vi "JSONtoLV-DBInsert.vi"(8 "error in":errorcluster, 11 "Output JSON Object":string) -> (0 "error out":errorcluster, 3 "value":T1)   [LabVIEW 2013]
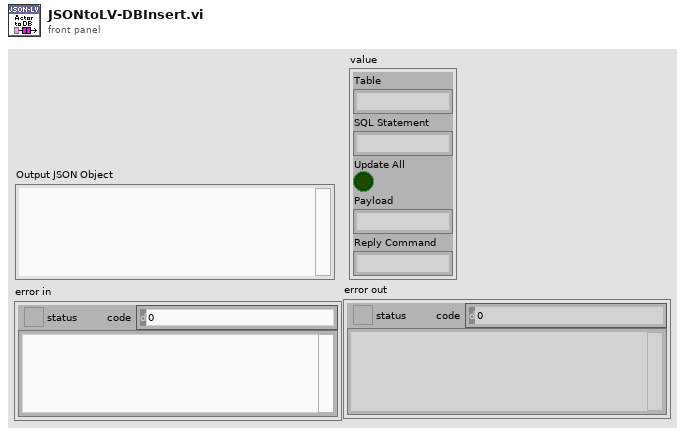
[diagram p1: front panel]
types:
  T1 = cluster{"Table":string, "SQL Statement":string, "Update All":bool, "Payload":string, "Reply Command":string}
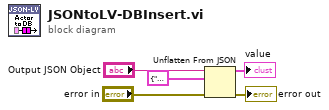
[diagram p0: block diagram]
diagram:
  n1 = Unflatten From JSON(JSON string="Output JSON Object", type and defaults=T1 {"Table"="", "SQL Statement"="", "Update All"=FALSE, "Payload"="", "Reply Command"=""} ("output cluster"), error in (no error)="error in") -> (value=→"value":T1, error out=→"error out":errorcluster)  [unwired: 4 in]
